vi "Add Operations.vi"(8 "error in (no error)":errorcluster caption="entrée d'erreur (pas d'erreur)", 10 "Added Operation":refnum<class "Operation.lvclass">, 11 "Operations en entrée":refnum<class "Operations.lvclass"> caption="DNL_LabVIEW Object in") -> (0 "error out":errorcluster caption="sortie d'erreur", 1 "created new?":bool, 3 "Operations en sortie":refnum<class "Operations.lvclass"> caption="DNL_LabVIEW Object out")   [LabVIEW 2012, in "Operations.lvclass"]
uses:
  Operations.lvclass
  Operation/Operation.lvclass
  <userlib>/_OpenG.lib/dictionary/dictionary.llb/Dictionary Key Value Pair Cluster__ogtk.ctl
  Operations.lvclass/Operations.ctl
  Operation/Operation.lvclass/Operation.ctl
  <userlib>/_OpenG.lib/dictionary/dictionary.llb/Dictionary Update (by scalar value)__ogtk.vi
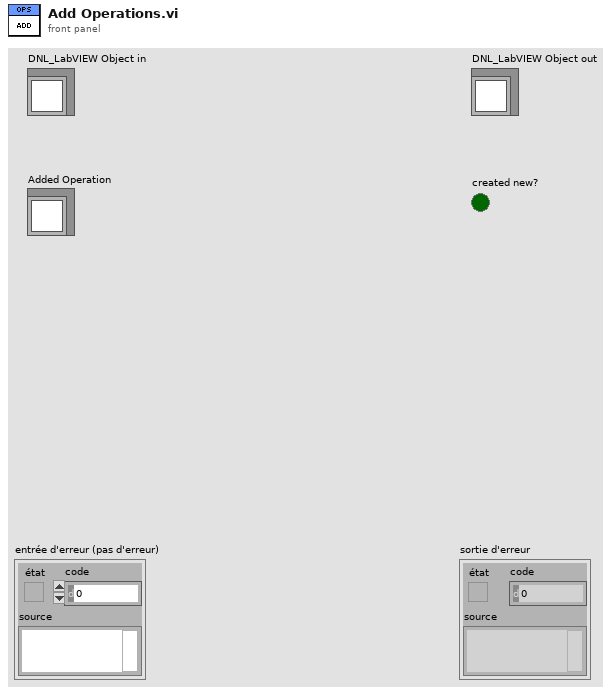
[diagram p1: front panel]
types:
  T1 = typedef "Dictionary Key Value Pair Cluster__ogtk.ctl" = cluster{"key":variant, "value":variant}
  T2 = typedef "Dictionary Object RefNum__ogtk.ctl" = refnum<k1>
  T3 = typedef "Operation Parameters.ctl" = cluster{"Date":timestamp, "Operation Type":T4, "Amount":dbl, "Comment":string, "Currency":T5}
  T4 = typedef "Operation Type Enum.ctl" = enum16{"Coupons", "Dépot", "Retrait", "Intérêts", "Taxe"}
  T5 = typedef "Currencies.ctl" = enum16{"Euro", "Dollar", "Yen", "RIM", "CHF"}
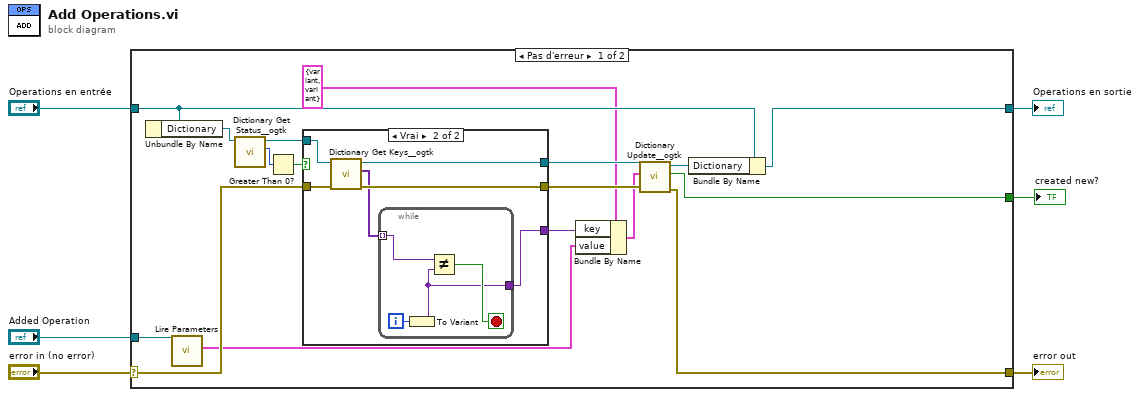
[diagram p0: block diagram]
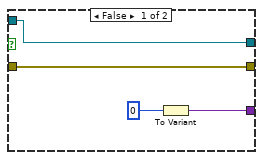
[diagram p2: hidden frame]
diagram:
  n1 = case shown="Pas d'erreur" "error in (no error)" {
    selector: "error in (no error)" -> [w17 w39]
    tunnel: [w20 w39] -> w5
    tunnel: [w22 w38] -> w3
    tunnel: "Operations en entrée" -> [w23 w38]
    tunnel: [w19 _] -> w2
    tunnel: "Added Operation" -> [w13 _]
    frame No Error {
      n2 = Unbundle By Name(w23) -> ("Dictionary"=w11:T2)
      n3 = call "Lire Parameters.vi"("Operation en entrée"=w13) -> ("Parameters"=w12:T3)  [unwired: 9 in, 1 out]
      n4 = call <userlib>:"Dictionary Get Status__ogtk.vi"("dictionary"=w11) -> ("size"=w10:i32, "dictionary out"=w9:T2)  [unwired: 8 in, 1 out]
      n5 = Greater Than 0?(x=w10) -> (x > 0?=w8:bool)
      n6 = case shown="Vrai" w8 {
        tunnel: [w24 w33] -> w18
        tunnel: w17 -> [w25 w32]
        tunnel: [w25 w31] -> w16
        tunnel: w9 -> [w24 w29]
        tunnel: [w26 w28] -> w7
        frame False {
          n7 = To Variant(anything=0 ("size")) -> (Variant=w26:variant)
        }
        frame True {
          n8 = call <userlib>:"Dictionary Get Keys__ogtk.vi"("error in (no error)"=w32, "dictionary"=w29) -> ("error out"=w31:errorcluster, "keys"=w30:variant[], "dictionary out"=w33:T2)  [unwired: 7 in]
          n9 = while {
            tunnel: w30 -> [w36] mode=indexing
            tunnel: [w34] -> w28
            i -> [w37]
            stop <- w35 stop-if-true
            n10 = To Variant(anything=w37) -> (Variant=w34:variant)
            n11 = Not Equal?(x=w36, y=w34) -> (x != y?=w35:bool)
          }
        }
      }
      n12 = Bundle By Name(cluster=T1 {"key"=variant, "value"=variant} ("key-value"), "key"=w7, "value"=w12) -> (w14:T1)
      n13 = call-poly <userlib>:"Dictionary Update__ogtk.vi"("error in (no error)"=w16, "key-value"=w14, "dictionary"=w18) -> ("error out"=w20:errorcluster, "created new?"=w19:bool, "dictionary out"=w21:T2)  [unwired: 6 in]
      n14 = Bundle By Name(cluster=w23, "Dictionary"=w21) -> (w22:refnum<class "Operations.lvclass">)
    }
    frame Error {
    }
  }
  "error out" <- w5
  "Operations en sortie" <- w3
  "created new?" <- w2
